vi "reset.vi"(8 "error in (no error)":errorcluster, 11 "Test Redis Client in":refnum<class "Test Redis Client.lvclass">) -> (0 "error out":errorcluster, 1 "remaining receive elements":string[](array[string]), 2 "remaining send elements":string[](array[string]), 3 "Test Redis Client out":refnum<class "Test Redis Client.lvclass">)   [LabVIEW 2019, in "Test Redis Client for LabVIEW.lvlib" / "Test Redis Client.lvclass"]
uses:
  Test Redis Client.lvclass
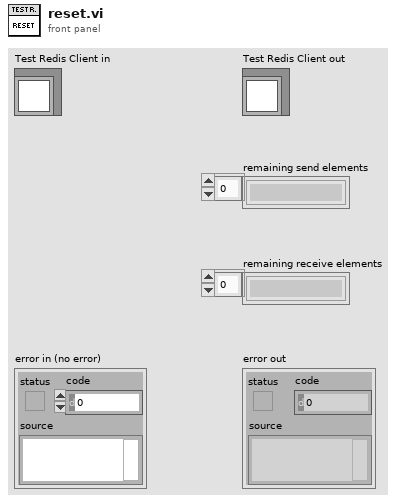
[diagram p1: front panel]
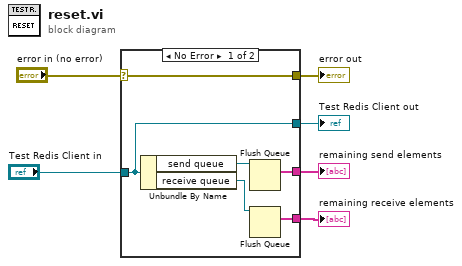
[diagram p0: block diagram]
diagram:
  n1 = case shown="No Error" "error in (no error)" {
    selector: "error in (no error)" -> [w12 w14]
    tunnel: [w12 w14] -> w5
    tunnel: [w11 w13] -> w3
    tunnel: "Test Redis Client in" -> [w11 w13]
    tunnel: [w8 _] -> w2
    tunnel: [w7 _] -> w1
    frame No Error {
      n2 = Unbundle By Name(w11) -> ("send queue"=w10:refnum<queue>, "receive queue"=w9:refnum<queue>)
      n3 = Flush Queue(queue=w10) -> (remaining elements=w8:string[])  [unwired: 1 in, 2 out]
      n4 = Flush Queue(queue=w9) -> (remaining elements=w7:string[])  [unwired: 1 in, 2 out]
    }
    frame Error {
    }
  }
  "error out" <- w5
  "Test Redis Client out" <- w3
  "remaining send elements" <- w2
  "remaining receive elements" <- w1
